vi "Load Theme - Light Gray.vi"(8 "error in (no error)":errorcluster) -> (0 "error out":errorcluster, 3 "Theme out":refnum<class "Theme.lvclass">)   [LabVIEW 2021, in "Theme.lvclass"]
doc: "Load the default light theme for pop ups\n\n<b>Code Developed By:</b> +\nDaniel Coons +\nhttps://github.com/danielcoons/tsc-pop-up"
uses:
  Theme.lvclass
  Dialog colors--typedef.ctl
  Button colors--typedef.ctl
  message box--typdef.ctl
  Theme.lvclass/Theme.ctl
  Popup/PopUp Theme Global.vi
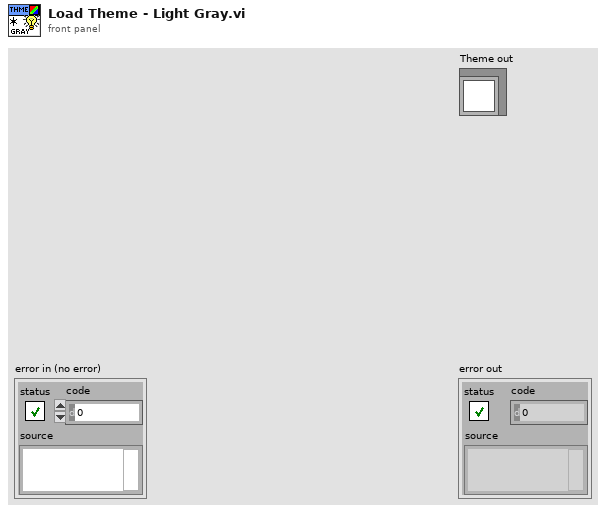
[diagram p1: front panel]
types:
  T1 = typedef "Theme.lvclass/message box--typdef.ctl" = cluster{"Text.Font Name":string, "Text.Font Size":u32, "Color":u32, "Text.Justification":enum16{"Left", "Center", "Right"}, "messge color":cluster{"border":u32, "fill":u32}}
  T2 = typedef "Theme.lvclass/Button colors--typedef.ctl" = cluster{"false color":cluster{"border":u32, "fill":u32}, "hover color":cluster{"border":u32, "fill":u32}, "press color":cluster{"border":u32, "fill":u32}, "Boolean Text":u32, "Text.Font Name":string, "Text.Font Size":u32, "Bold?":bool, "Itallic?":bool}
  T3 = typedef "Theme.lvclass/Dialog colors--typedef.ctl" = cluster{"Header":u32, "Background":u32, "Picture Background":u32}
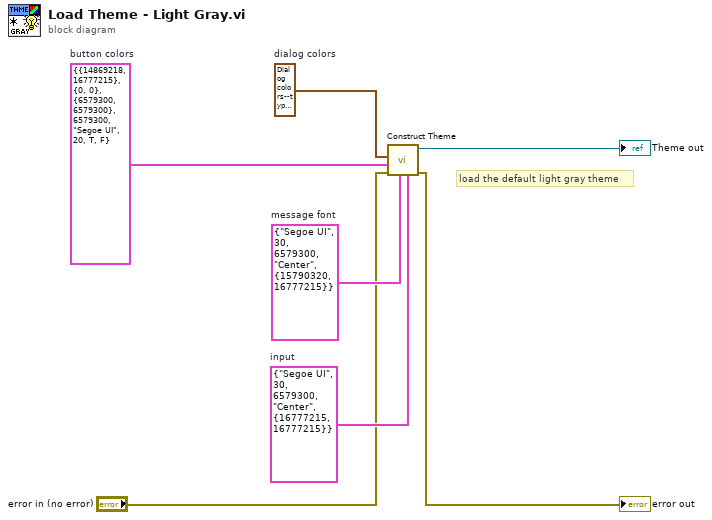
[diagram p0: block diagram]
diagram:
  w4 = T1 {"Text.Font Name"="Segoe UI", "Text.Font Size"=30, "Color"=6579300, "Text.Justification"=enum."Center", "messge color"={"border"=16777215, "fill"=16777215}}  # input
  w5 = T1 {"Text.Font Name"="Segoe UI", "Text.Font Size"=30, "Color"=6579300, "Text.Justification"=enum."Center", "messge color"={"border"=15790320, "fill"=16777215}}  # message font
  w6 = T2 {"false color"={"border"=14869218, "fill"=16777215}, "hover color"={"border"=0, "fill"=0}, "press color"={"border"=6579300, "fill"=6579300}, "Boolean Text"=6579300, "Text.Font Name"="Segoe UI", "Text.Font Size"=20, "Bold?"=TRUE, "Itallic?"=FALSE}  # button colors
  w7 = T3 {"Header"=11579568, "Background"=15790320, "Picture Background"=16777216}  # dialog colors
  # "load the default light gray theme"
  n1 = call "Construct Theme.vi"("input"=w4, "message font"=w5, "error in (no error)"="error in (no error)", "button colors"=w6, "dialog colors"=w7) -> ("error out"=→"error out":errorcluster, "Theme out"=→"Theme out":refnum<class "Theme.lvclass">)  [unwired: 5 in]
